vi "Get DDS Cur Boxing Bias Mv Min.vi"(8 "error in (no error)":errorcluster, 11 "boxing":u32) -> (0 "error out":errorcluster, 3 "function return":i32)   [LabVIEW 2021, in "vmmso.lvlib"]
doc: "DLL_API int WINAPI GetDDSCurBoxingBiasMvMin(unsigned int boxing);"
uses:
  vmmso.lvlib
  vmmso.dll
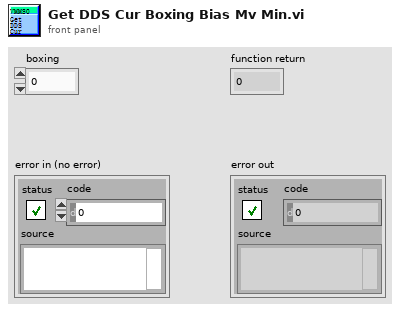
[diagram p1: front panel]
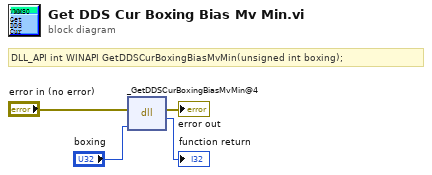
[diagram p0: block diagram]
diagram:
  # "DLL_API int WINAPI GetDDSCurBoxingBiasMvMin(unsigned int boxing);"
  n1 = dll-call lib="O:/MSO/library/demo-Labview/vmmso/vmmso.*" fn="_GetDDSCurBoxingBiasMvMin@4"(error in="error in (no error)", "boxing"="boxing") -> (error out=→"error out":errorcluster, →"function return":i32)  [unwired: 3 in, 1 out]
